vi "RingsToIni.vi"(8 "ErrorArray in":errorcluster[](array[cluster]), 10 "RingRefArray":refnum<vi>[](array[refnum]), 11 "IniFileRef in":T1) -> (0 "ErrorArray out":errorcluster[](array[cluster]), 3 "InifileRef out":T1)   [LabVIEW 2014, in "Ini_lib.lvlib"]
uses:
  <vilib>/Utility/config.llb/Config Data RefNum.ctl
  Ini_lib.lvlib
  <userlib>/NIST/NISTErrorLib/NISTErrorLib.lvlib
  <vilib>/Utility/config.llb/NI_LVConfig.lvlib
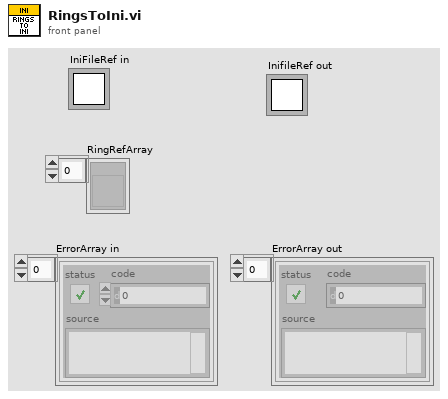
[diagram p1: front panel]
types:
  T1 = typedef "NI_LVConfig.lvlib/Config Data RefNum.ctl" = refnum<k1>
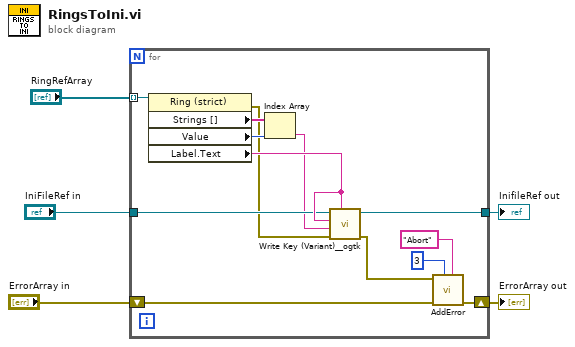
[diagram p0: block diagram]
diagram:
  n1 = for {
    tunnel: "RingRefArray" -> [w18] mode=indexing
    tunnel: "IniFileRef in" -> [w16]
    shift-right: [w9] -> w4
    shift-left: "ErrorArray in" -> [w10]
    tunnel: [w8] -> w2
    n2 = property class="Ring (strict)"(reference=w18) -> (error out=w6:errorcluster, "Strings []"=w15:string[], "Value"=w14:u16, "Label.Text"=w17:string)  [unwired: 1 in, 1 out]
    n3 = Index Array(array=w15, index=w14) -> (element=w13:string)
    n4 = call <userlib>:"Write Key (Variant)__ogtk.vi"("section"=w17, "error in (no error)"=w6, "key-value"=w13, "key (optional)"=w17, "refnum"=w16) -> ("error out"=w7:errorcluster, "refnum out"=w8:T1)  [unwired: 5 in]
    n5 = call <userlib>:"AddError.vi"("Severity"="Abort", "Priority"=u8 3, "ErrorArray"=w10, "error in (no error)"=w7) -> ("ErrorArray"=w9:errorcluster[])  [unwired: 6 in, 1 out]
  }
  "ErrorArray out" <- w4
  "InifileRef out" <- w2
